vi "Add Permissions.vi"(8 "error in (no error)":errorcluster, 9 "Accounts and Actions":T1[](array[typedef]), 10 "Label":string, 11 "SQS in":refnum<class "NI_AWS_SQS.lvclass">) -> (0 "error out":errorcluster, 3 "SQS out":refnum<class "NI_AWS_SQS.lvclass">)   [LabVIEW 2015, in "NI_AWS_SQS.lvclass"]
uses:
  NI_AWS_SQS.lvclass
  Account and Action.ctl
  Permission Action.ctl
  Core/Name Value Pair.ctl
  Core/Request Options.ctl
  NI_AWS_SQS.lvclass/NI_AWS_SQS.ctl
  Read Account Number.vi
  Read Name.vi
  Core/NI_AWS_Core.lvclass
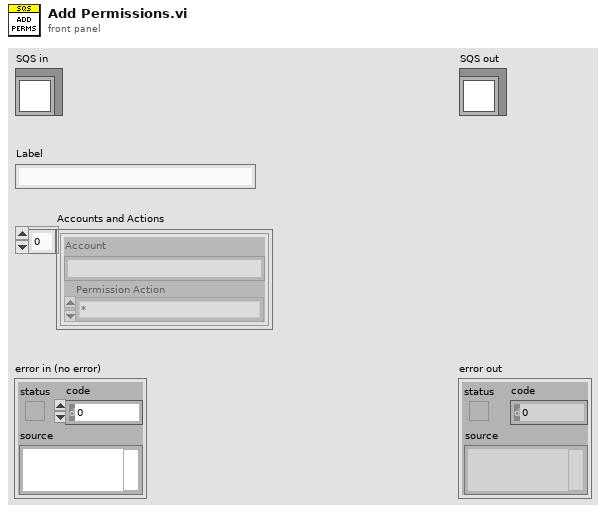
[diagram p1: front panel]
types:
  T1 = typedef "NI_AWS_SQS.lvclass/Account and Action.ctl" = cluster{"Account":string, "Permission Action":T2}
  T2 = typedef "NI_AWS_SQS.lvclass/Permission Action.ctl" = enum16{"*", "ChangeMessageVisibility", "DeleteMessage", "GetQueueAttributes", "GetQueueUrl", "ReceiveMessage", "SendMessage"}
  T3 = typedef "NI_AWS_Core.lvclass/Name Value Pair.ctl" = cluster{"name":string, "value":string}
  T4 = typedef "NI_AWS_Core.lvclass/Request Options.ctl" = cluster{"request headers":T3[], "request parameters":T3[], "request body":string}
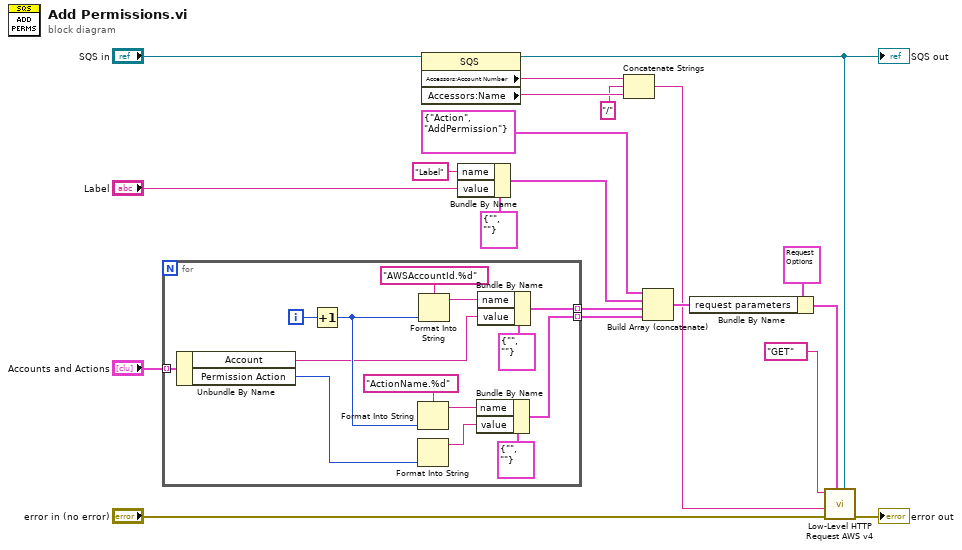
[diagram p0: block diagram]
diagram:
  n1 = for {
    tunnel: "Accounts and Actions" -> [w29] mode=indexing
    tunnel: [w30] -> w16 mode=indexing
    tunnel: [w25] -> w12 mode=indexing
    i -> [w34]
    n2 = Unbundle By Name(w29) -> ("Account"=w23:string, "Permission Action"=w22:T2)
    n3 = Increment(x=w34) -> (x+1=w24:i32)
    n4 = Format Into String(format string="ActionName.%d", w24) -> (resulting string=w28:string)  [unwired: 2 in, 1 out]
    n5 = Format Into String(w22) -> (resulting string=w21:string)  [unwired: 3 in, 1 out]
    n6 = Format Into String(format string="AWSAccountId.%d", w24) -> (resulting string=w31:string)  [unwired: 2 in, 1 out]
    n7 = Bundle By Name(cluster=T3 {"name"="", "value"=""} ("element"), "name"=w28, "value"=w21) -> (w25:T3)
    n8 = Bundle By Name(cluster=T3 {"name"="", "value"=""} ("element"), "name"=w31, "value"=w23) -> (w30:T3)
  }
  n9 = property class="SQS"(reference="SQS in") -> (reference out=w10:refnum<class "NI_AWS_SQS.lvclass">, "Accessors:Account Number"=w15:string, "Accessors:Name"=w14:string)  [unwired: 1 in, 1 out]
  "SQS out" <- w10
  n10 = Bundle By Name(cluster=T3 {"name"="", "value"=""} ("element"), "name"="Label", "value"="Label") -> (w3:T3)
  n11 = Concatenate Strings(w15, "/", w14) -> (w6:string)
  n12 = Build Array (concatenate)(T3 {"name"="Action", "value"="AddPermission"} ("Cluster"), w3, w16, w12) -> (w17:T3[])
  n13 = Bundle By Name(cluster=T4 {"request headers"=[], "request parameters"=[{"name"="Action", "value"="ListQueues"}], "request body"=""} ("Request Options"), "request parameters"=w17) -> (w18:T4)
  n14 = call "Low-Level HTTP Request AWS v4.vi"("AWS Core"=w10, "Request Options"=w18, "error in (no error)"="error in (no error)", "URL Suffix"=w6, "HTTP-Verb"="GET") -> ("error out"=→"error out":errorcluster)  [unwired: 4 in, 2 out]
